vi "Clear DTC.vi"(6 "Action":T3, 8 "error in":errorcluster, 9 "Address (ALL)":string="ALL", 10 "Address Lookup Table":variant, 11 "connection info":T1) -> (0 "error out":errorcluster, 2 "Address Lookup Table Out":variant, 3 "connection info":T1)   [LabVIEW 2015, in "J1939 Host Automation API.lvlib"]
uses:
  J1939 Host Automation API.lvlib
  <vilib>/NI/STM/TCP/TCP Connection Info.ctl
  <vilib>/NI/STM/SubVIs/MetaDataElement.ctl
  Types/DTC_Action.ctl
  Shared/J1939 Addon Shared.lvlib
  <vilib>/NI/STM/NI STM.lvlib
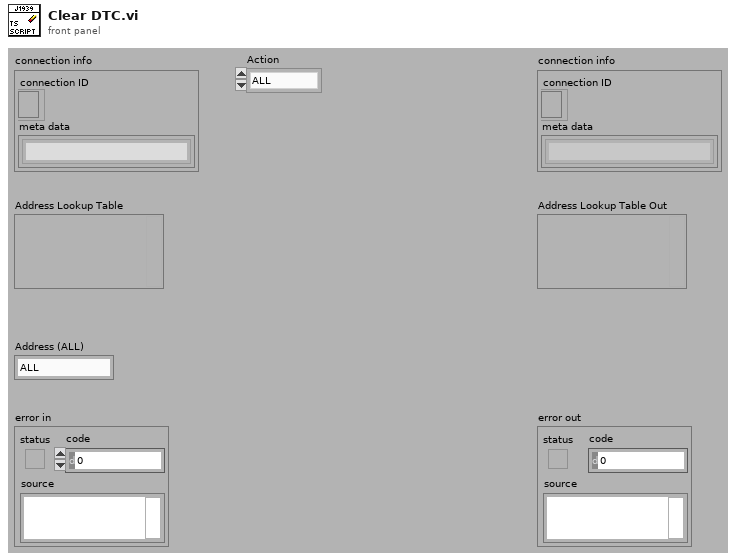
[diagram p1: front panel]
types:
  T1 = typedef "NI STM.lvlib/TCP Connection Info.ctl" = cluster{"connection ID":refnum<k5>, "meta data":T2[]}
  T2 = typedef "NI STM.lvlib/MetaDataElement.ctl" = string
  T3 = typedef "J1939 Host Automation API.lvlib/DTC_Action.ctl" = enum16{"ALL", "ACTIVE", "INACTIVE"}
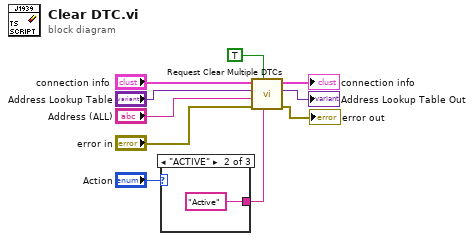
[diagram p0: block diagram]
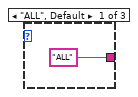
[diagram p2: hidden frame]
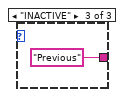
[diagram p3: hidden frame]
diagram:
  n1 = case shown="\"ACTIVE\"" "Action" {
    tunnel: ["ALL" ("TLA (ALL)") "Active" ("TLA (ALL)") "Previous" ("TLA (ALL)")] -> w5
    frame "ALL", Default {
    }
    frame "ACTIVE" {
    }
    frame "INACTIVE" {
    }
  }
  n2 = call "Request Clear Multiple DTCs.vi"("Command"=w5, "Ignore Response"=TRUE, "error in"="error in", "Address"="Address (ALL)", "Lookup Table"="Address Lookup Table", "connection info"="connection info") -> ("error out"=→"error out":errorcluster, "Lookup Table"=→"Address Lookup Table Out":variant, "connection info"=→"connection info":T1)  [unwired: 2 in, 1 out]
